vi "for_l0.vi"() -> ()   [LabVIEW 2010]
panel:
  out "Waveform Graph":dbl[](graph)=[1.0, 1.0, 1.0, 1.0, 1.0, 1.0, 1.0, 1.0, 1.0, 1.0, 1.0, 1.0, 1.0, 1.0, 1.0, 1.0, 1.0, 0.0, 0.0, 0.0, 1.0, 1.0, 1.0, 1.0, 1.0, 1.0, 1.0, 1.0, 1.0, 1.0, 1.0, 1.0, 1.0, 1.0, 1.0, 1.0, 1.0, 0.0, 0.0, 0.0, 1.0, 1.0, 1.0, 1.0, 1.0, 1.0, 1.0, 1.0, 1.0, 1.0, 1.0, 1.0, 1.0, 1.0, 1.0, 1.0, 1.0, 0.0, 0.0, 0.0, 1.0, 1.0, 1.0, 1.0, 1.0, 1.0, 1.0, 1.0, 1.0, 1.0, 1.0, 1.0, 1.0, 1.0, 1.0, 1.0, 1.0, 0.0, 0.0, 0.0]
  in  "stop":bool
  in  "Width":dbl(slide)=17.48768472906404 scale=0.0..20.0
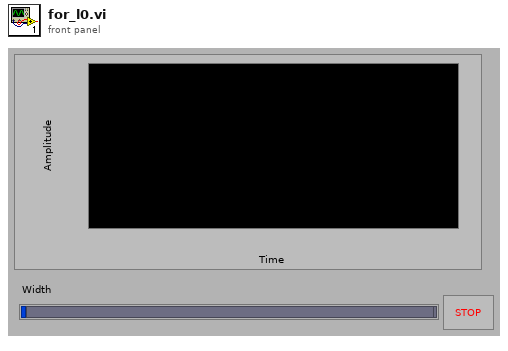
[diagram p1: front panel]
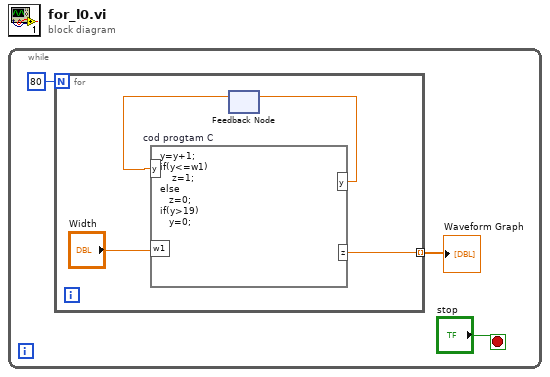
[diagram p0: block diagram]
diagram:
  n1 = while {
    stop <- "stop" stop-if-true
    n2 = for {
      N: 80 -> [_]
      tunnel: [w7] -> w1 mode=indexing
      n3 = feedback #1() -> (w5:dbl)  [unwired: 1 in]
      n4 = formula code="y=y+1;\nif(y<=w1)\n    z=1;\nelse\n   z=0;\nif(y>19)\n   y=0;" "cod progtam C"("w1"="Width", "y"=w5) -> ("z"=w7:dbl, "y"=w6:dbl)
      n5 = feedback-in #1(w6) -> ()
    }
    "Waveform Graph" <- w1
  }
